vi "make_stage_array (SubVI).vi"(11 "Stage settings:":T1) -> (3 "Tot Stage Arr":dbl[][](array[numeric]))   [LabVIEW 2014]
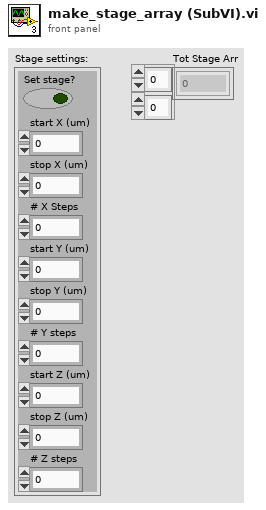
[diagram p1: front panel]
types:
  T1 = cluster{"Set stage?":bool, "start X (um)":ext, "stop X (um) ":ext, "# X Steps":i32, "start Y (um)":ext, "stop Y (um) ":ext, "# Y steps":i32, "start Z (um)":ext, "stop Z (um)":ext, "# Z steps ":i32}
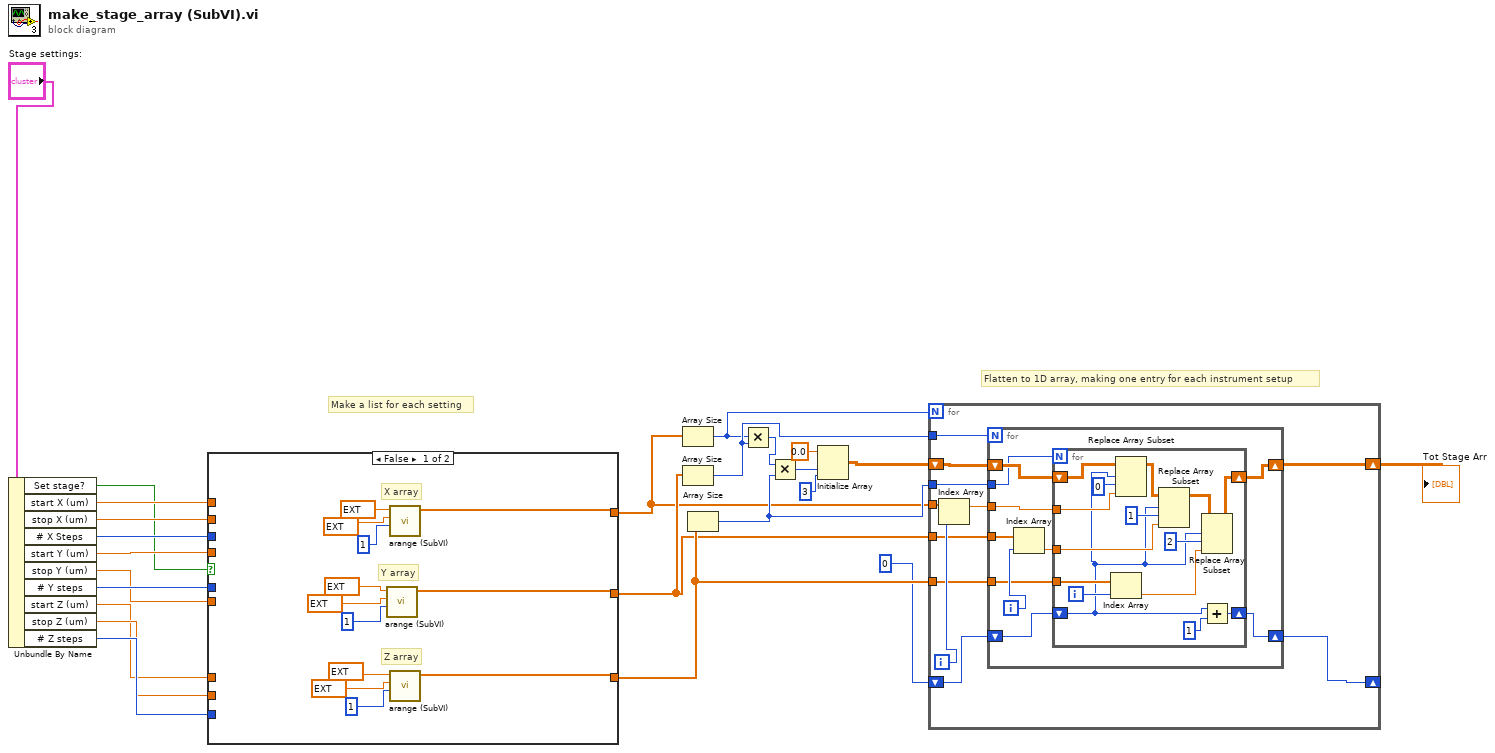
[diagram p0: block diagram]
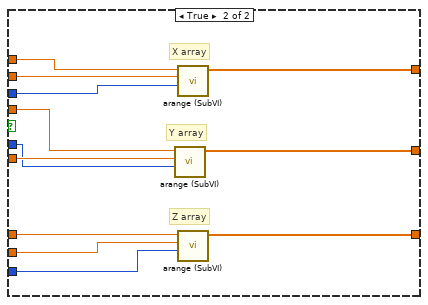
[diagram p2: hidden frame]
diagram:
  # "Make a list for each setting"
  # "Flatten to 1D array, making one entry for each instrument setup"
  n1 = Unbundle By Name("Stage settings:") -> ("Set stage?"=w1:bool, "start X (um)"=w2:ext, "stop X (um)"=w3:ext, "# X Steps"=w4:i32, "start Y (um)"=w5:ext, "stop Y (um)"=w6:ext, "# Y steps"=w7:i32, "start Z (um)"=w8:ext, "stop Z (um)"=w9:ext, "# Z steps"=w10:i32)
  n2 = case shown="False" w1 {
    tunnel: w2 -> [_ w48]
    tunnel: w3 -> [_ w47]
    tunnel: w4 -> [_ w46]
    tunnel: w5 -> [_ w45]
    tunnel: w6 -> [_ w44]
    tunnel: w7 -> [_ w43]
    tunnel: w8 -> [_ w42]
    tunnel: w9 -> [_ w41]
    tunnel: w10 -> [_ w40]
    tunnel: [w27 w39] -> w18
    tunnel: [w26 w38] -> w19
    tunnel: [w25 w37] -> w20
    frame False {
      # "Z array"
      # "Y array"
      # "X array"
      n3 = call "arange (SubVI).vi"("# Steps"=1, "stop"=ext -9999.0, "start"=ext -9999.0) -> ("Array"=w26:ext[])  [unwired: 8 in]
      n4 = call "arange (SubVI).vi"("# Steps"=1, "stop"=ext -9999.0, "start"=ext -9999.0) -> ("Array"=w27:ext[])  [unwired: 8 in]
      n5 = call "arange (SubVI).vi"("# Steps"=1, "stop"=ext -9999.0, "start"=ext -9999.0) -> ("Array"=w25:ext[])  [unwired: 8 in]
    }
    frame True {
      # "Z array"
      # "Y array"
      # "X array"
      n6 = call "arange (SubVI).vi"("# Steps"=w43, "stop"=w44, "start"=w45) -> ("Array"=w38:ext[])  [unwired: 8 in]
      n7 = call "arange (SubVI).vi"("# Steps"=w46, "stop"=w47, "start"=w48) -> ("Array"=w39:ext[])  [unwired: 8 in]
      n8 = call "arange (SubVI).vi"("# Steps"=w40, "stop"=w41, "start"=w42) -> ("Array"=w37:ext[])  [unwired: 8 in]
    }
  }
  n9 = Array Size(array=w18) -> (size(s)=w21:i32)
  n10 = Array Size(array=w19) -> (size(s)=w22:i32)
  n11 = Array Size(array=w20) -> (size(s)=w23:i32)
  n12 = Multiply(x=w21, y=w22) -> (x*y=w12:i32)
  n13 = Multiply(x=w12, y=w23) -> (x*y=w13:i32)
  n14 = Initialize Array(0.0 ("element"), w13, 3 ("dimension size")) -> (w15:dbl[][])
  n15 = for {
    N: w21 -> [_]
    shift-right: [w49] -> _
    shift-left: 0 ("disabled index (row)") -> [w50]
    shift-right: [w58] -> w17
    shift-left: w15 -> [w59]
    tunnel: w18 -> [w57]
    tunnel: w19 -> [w54]
    tunnel: w20 -> [w53]
    tunnel: w22 -> [w52]
    tunnel: w23 -> [w51]
    i -> [w55]
    n16 = Index Array(array=w57, index=w55) -> (element=w56:ext)
    n17 = for {
      N: w52 -> [_]
      tunnel: w56 -> [w67]
      tunnel: w54 -> [w66]
      tunnel: w53 -> [w63]
      tunnel: w51 -> [w62]
      shift-right: [w68] -> w58
      shift-left: w59 -> [w69]
      shift-right: [w60] -> w49
      shift-left: w50 -> [w61]
      i -> [w65]
      n18 = Index Array(array=w66, index=w65) -> (element=w64:ext)
      n19 = for {
        N: w62 -> [_]
        tunnel: w67 -> [w77]
        tunnel: w64 -> [w76]
        tunnel: w63 -> [w74]
        shift-right: [w80] -> w68
        shift-left: w69 -> [w84]
        shift-right: [w71] -> w60
        shift-left: w61 -> [w70]
        i -> [w75]
        n20 = Index Array(array=w74, index=w75) -> (element=w73:ext)
        n21 = Replace Array Subset(array=w84, new element=w77, index (row)=w70, index (col)=0 ("disabled index (col)")) -> (w82:dbl[][])
        n22 = Replace Array Subset(array=w82, new element=w76, index (row)=w70, index (col)=1 ("disabled index (col)")) -> (w81:dbl[][])
        n23 = Replace Array Subset(array=w81, new element=w73, index (row)=w70, index (col)=2 ("disabled index (col)")) -> (w80:dbl[][])
        n24 = Add(x=w70, y=1) -> (x+y=w71:i32)
      }
    }
  }
  "Tot Stage Arr" <- w17
